vi "Apply Decryption Transformation.vi"(8 "error in (no error)":errorcluster, 10 "Encrypted data in":u8[](array[numeric]), 11 "Crypto transform in":refnum<k24>) -> (0 "error out":errorcluster, 2 "Plaintext":u8[](array[numeric]), 3 "Crypto transform out":refnum<k24>)   [LabVIEW 2021, in "dotNET Crypto Symmetric Encryption.lvlib"]
doc: "Decrypt text using the supplied .NET CryptoTransform object."
uses:
  dotNET Crypto Symmetric Encryption.lvlib
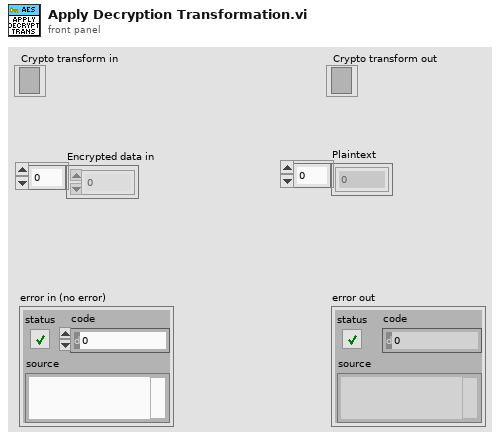
[diagram p1: front panel]
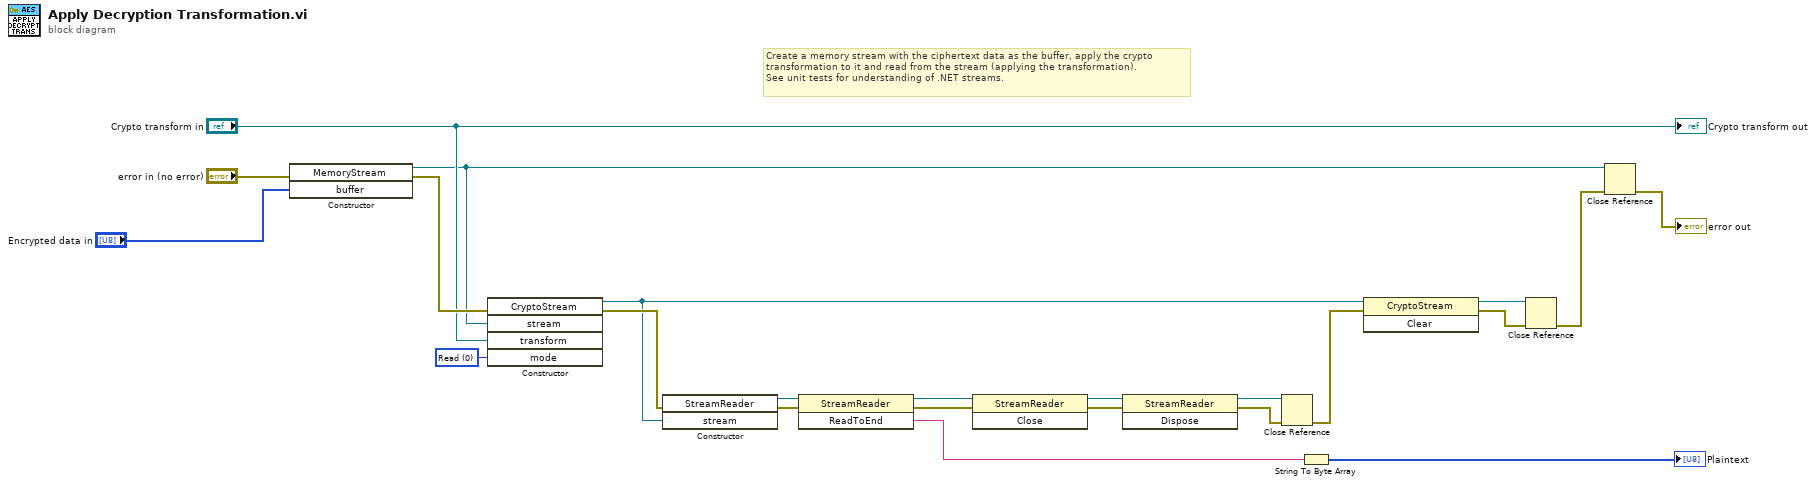
[diagram p0: block diagram]
diagram:
  w8 = 0 items=["Read", "Write"] ("mode")
  # "Create a memory stream with the ciphertext data as the buffer, apply the crypto transformation to it and read from the stream (applying the transformation).\nSee unit tests for understanding of .NET streams."
  n1 = constructor class="MemoryStream"(error in="error in (no error)", "buffer"="Encrypted data in") -> (reference out=w10:refnum<k24>, error out=w16:errorcluster)  [unwired: 2 in, 2 out]
  n2 = constructor class="CryptoStream"(error in=w16, "stream"=w10, "transform"="Crypto transform in", "mode"=w8) -> (reference out=w21:refnum<k24>, error out=w23:errorcluster)  [unwired: 2 in, 4 out]
  n3 = constructor class="StreamReader"(error in=w23, "stream"=w21) -> (reference out=w22:refnum<k24>, error out=w20:errorcluster)  [unwired: 2 in, 2 out]
  n4 = invoke class="StreamReader" method="ReadToEnd"(reference=w22, error in=w20) -> (reference out=w9:refnum<k24>, error out=w13:errorcluster, "ReadToEnd"=w19:string)  [unwired: 1 in]
  n5 = invoke class="StreamReader" method="Close"(reference=w9, error in=w13) -> (reference out=w5:refnum<k24>, error out=w4:errorcluster)  [unwired: 1 in, 1 out]
  n6 = invoke class="StreamReader" method="Dispose"(reference=w5, error in=w4) -> (reference out=w2:refnum<k24>, error out=w3:errorcluster)  [unwired: 1 in, 1 out]
  n7 = Close Reference(reference=w2, error in (no error)=w3) -> (error out=w14:errorcluster)
  n8 = String To Byte Array(string=w19) -> (unsigned byte array=→"Plaintext":u8[])
  n9 = invoke class="CryptoStream" method="Clear"(reference=w21, error in=w14) -> (reference out=w6:refnum<k24>, error out=w7:errorcluster)  [unwired: 1 in, 1 out]
  n10 = Close Reference(reference=w6, error in (no error)=w7) -> (error out=w15:errorcluster)
  n11 = Close Reference(reference=w10, error in (no error)=w15) -> (error out=→"error out":errorcluster)
  "Crypto transform out" <- "Crypto transform in"
